vi "Abort Sub2.vi"(11 "Test Case In":refnum<class "Tests Event MessengerM.lvclass">) -> (0 "error out":errorcluster, 3 "Test Case Out":refnum<class "Tests Event MessengerM.lvclass">)   [LabVIEW 2020, in "Tests Event MessengerM.lvclass"]
uses:
  Tests Event MessengerM.lvclass
  Tests Event MessengerM.lvclass/Tests Event MessengerM.ctl
  C:/Program Files/National Instruments/LabVIEW 2026/vi.lib/Astemes/LUnit/Test Case.lvclass
  C:/Program Files/National Instruments/LabVIEW 2026/vi.lib/Astemes/LUnit/LUnit Runnable.lvclass
  D:/git/Event-MessengerM-Channel-Wire/tests/Tests Event MessengerM/Tests Event MessengerM.lvclass
  <vilib>/Astemes/LUnit/Test Case.lvclass
  8a53ca5d-0537-4ac6-b774-ad5cdbdca4c7.vi
  e96872dd-892a-43da-91d9-4e6e3ca0f4e8.vi
  fa70241b-6bb2-40b9-9a1d-70773653dfce.vi
  91f61d9e-5a40-4597-ae06-be44812c59d4.vi
  2eb94fc6-1cac-487b-95ad-6a276148d9d0.vi
panel:
  out "cmd 2":string
  out "cmd":string
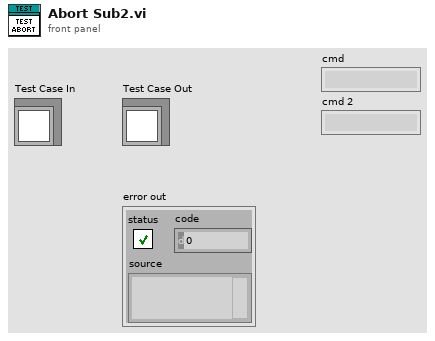
[diagram p1: front panel]
types:
  T1 = typedef "Event MessengerM-c(str,var).lvlib/))Channel.ctl" = refnum<queue>
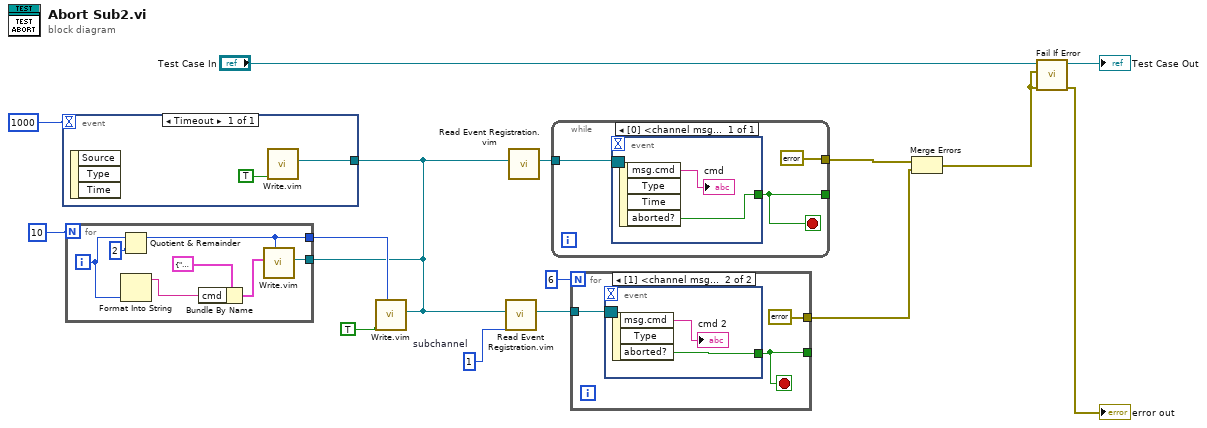
[diagram p0: block diagram]
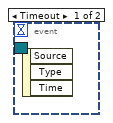
[diagram p2: hidden frame]
diagram:
  w1 = 1  # subchannel
  n1 = for {
    N: 10 -> [_]
    tunnel: [w16] -> w5
    tunnel: [w17] -> w2
    i -> [w20]
    n2 = Quotient & Remainder(x=w20, y=2) -> (x-y*floor(x/y)=w16:i32)  [unwired: 1 out]
    n3 = Format Into String(w20) -> (resulting string=w19:string)  [unwired: 3 in, 1 out]
    n4 = Bundle By Name(cluster=cluster{"cmd":string, "data":variant} {"cmd"="", "data"=variant} ("element"), "cmd"=w19) -> (w18:cluster{"cmd":string, "data":variant})
    n5 = call "Write.vim"("subchannel"=w16, "element"=w18) -> ("channel"=w17:T1)  [unwired: 8 in, 1 out]
  }
  n6 = event shown="[0] Timeout" {
    selector: _ -> [_]
    dyn-events: _ -> [_]
    timeout: 1000 -> [_]
    tunnel: w2 -> [w23]
    event Timeout {
      n7 = event-data() -> ()  [unwired: 1 in, 3 out]
      n8 = call "Write.vim"("abort sub (F)"=TRUE) -> ("channel"=w23:T1)  [unwired: 9 in, 1 out]
    }
  }
  n9 = call "Write.vim"("channel"=w2, "subchannel"=w5, "abort sub (F)"=TRUE) -> ()  [unwired: 8 in, 1 out]
  n10 = call "Read Event Registration.vim"("subchannel"=w1, "channel"=w2) -> ("event registration refnum"=w4:refnum<event-registration>)  [unwired: 9 in]
  n11 = call "Read Event Registration.vim"("channel"=w2) -> ("event registration refnum"=w3:refnum<event-registration>)  [unwired: 10 in]
  n12 = while {
    tunnel: w3 -> [w27]
    tunnel: [w26] -> _
    tunnel: [errorcluster {"status"=FALSE, "code"=0, "source"=""} ("error constant")] -> w9
    stop <- w26 stop-if-true
    n13 = event shown="[0] <channel msg>: User Event" {
      selector: w27 -> [_]
      dyn-events: _ -> [_]
      timeout: _ -> [_]
      tunnel: [w28] -> w26
      event User Event {
        n14 = event-data() -> ("msg.cmd"=→"cmd":string, "aborted?"=w28:bool)  [unwired: 1 in, 2 out]
      }
    }
  }
  n15 = for {
    N: 6 -> [_]
    tunnel: w4 -> [w32]
    tunnel: [w31] -> _
    tunnel: [errorcluster {"status"=FALSE, "code"=0, "source"=""} ("error constant")] -> w8
    stop <- w31 stop-if-true
    n16 = event shown="[1] <channel msg>: User Event" {
      selector: w32 -> [_ _]
      dyn-events: _ -> [_ _]
      timeout: _ -> [_ _]
      tunnel: [_ w33] -> w31
      event Timeout {
        n17 = event-data() -> ()  [unwired: 1 in, 3 out]
      }
      event User Event {
        n18 = event-data() -> ("msg.cmd"=→"cmd 2":string, "aborted?"=w33:bool)  [unwired: 1 in, 1 out]
      }
    }
  }
  n19 = Merge Errors(w9, w8) -> (w7:errorcluster)
  n20 = call <vilib>:"Fail If Error.vi"("error in (no error)"=w7, "Assert error"=w7, "LUnit Test Case In"="Test Case In") -> ("error out"=→"error out":errorcluster, "LUnit Test Case Out"=→"Test Case Out":refnum<class "Tests Event MessengerM.lvclass">)  [unwired: 7 in]
